vi "GetRandomNum.vi"(8 "error in (no error)":errorcluster, 11 "Generator in":refnum<class "Generator.lvclass">) -> (0 "error out":errorcluster, 3 "Generator out":refnum<class "Generator.lvclass">)   [LabVIEW 2021, in "Generator.lvlib" / "Generator.lvclass"]
uses:
  Generator.lvclass
  Generator.lvclass/Generator.ctl
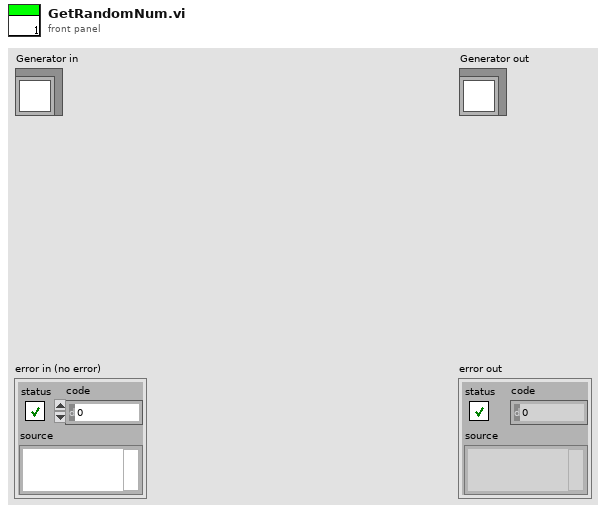
[diagram p1: front panel]
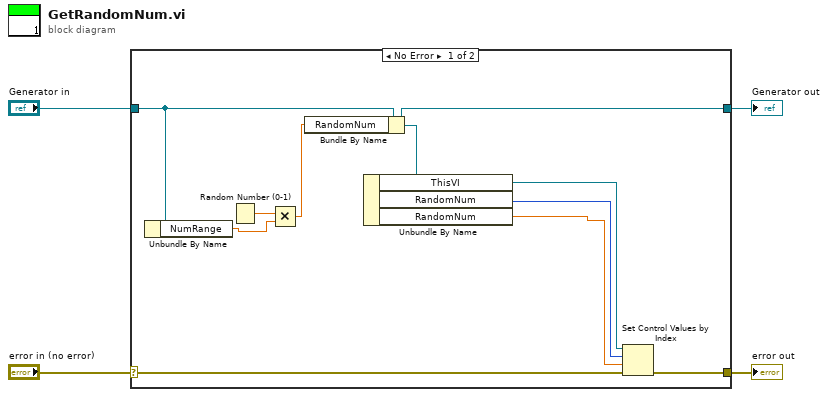
[diagram p0: block diagram]
diagram:
  n1 = case shown="No Error" "error in (no error)" {
    selector: "error in (no error)" -> [w14 w16]
    tunnel: [w9 w16] -> w3
    tunnel: [w8 w15] -> w1
    tunnel: "Generator in" -> [w11 w15]
    frame No Error {
      n2 = Unbundle By Name(w11) -> ("NumRange"=w10:dbl)
      n3 = Random Number (0-1)() -> (number: 0 to 1=w13:dbl)
      n4 = Multiply(x=w13, y=w10) -> (x*y=w12:dbl)
      n5 = Bundle By Name(cluster=w11, "RandomNum"=w12) -> (w8:refnum<class "Generator.lvclass">)
      n6 = Unbundle By Name(w8) -> ("ThisVI"=w7:refnum<vi>, "RandomNum"=w6:i32, "RandomNum"=w5:dbl)
      n7 = Set Control Values by Index(0:w7, 1:w6, 2:w5, 3:w14) -> (11:w9:errorcluster)
    }
    frame Error {
    }
  }
  "error out" <- w3
  "Generator out" <- w1
